vi "calibrate_handle.vi"(8 "Decimated pose (manipulator)":dbl[][][](array[numeric]) format="%#_3p", 9 "Tip offset":sgl[](array[numeric]), 11 "Light 3 pos":sgl[][](array[numeric])) -> (0 "Handle error":T1 format="%#_3g", 1 "RMS Error":dbl format="%#_3g", 3 "Handle transform":T1 format="%#_3p")   [LabVIEW 2013]
uses:
  <vilib>/Analysis/Matrix/Datatypes/RealMatrix.ctl
  <vilib>/Analysis/baseanly.llb/A x Vector.vi
  <vilib>/Analysis/baseanly.llb/Vector x A.vi
  <vilib>/Analysis/_algsub.llb/Real PseudoInverse Matrix.vi
  <vilib>/Analysis/baseanly.llb/Real A x B.vi
  <vilib>/Analysis/Matrix/Numeric/Multiply/Multiply - RM,RM.vi
  <vilib>/Analysis/NI_AALBase.lvlib
  <vilib>/Analysis/NI_AALPro.lvlib
  <vilib>/Analysis/Matrix/NI_Matrix.lvlib
panel:
  out "Calibrated central tip pos in manipulator":dbl[][](graph)
  out "L3 pos in manipulator":dbl[][](graph)
  out "Central tip pos in manipulator":dbl[][](graph)
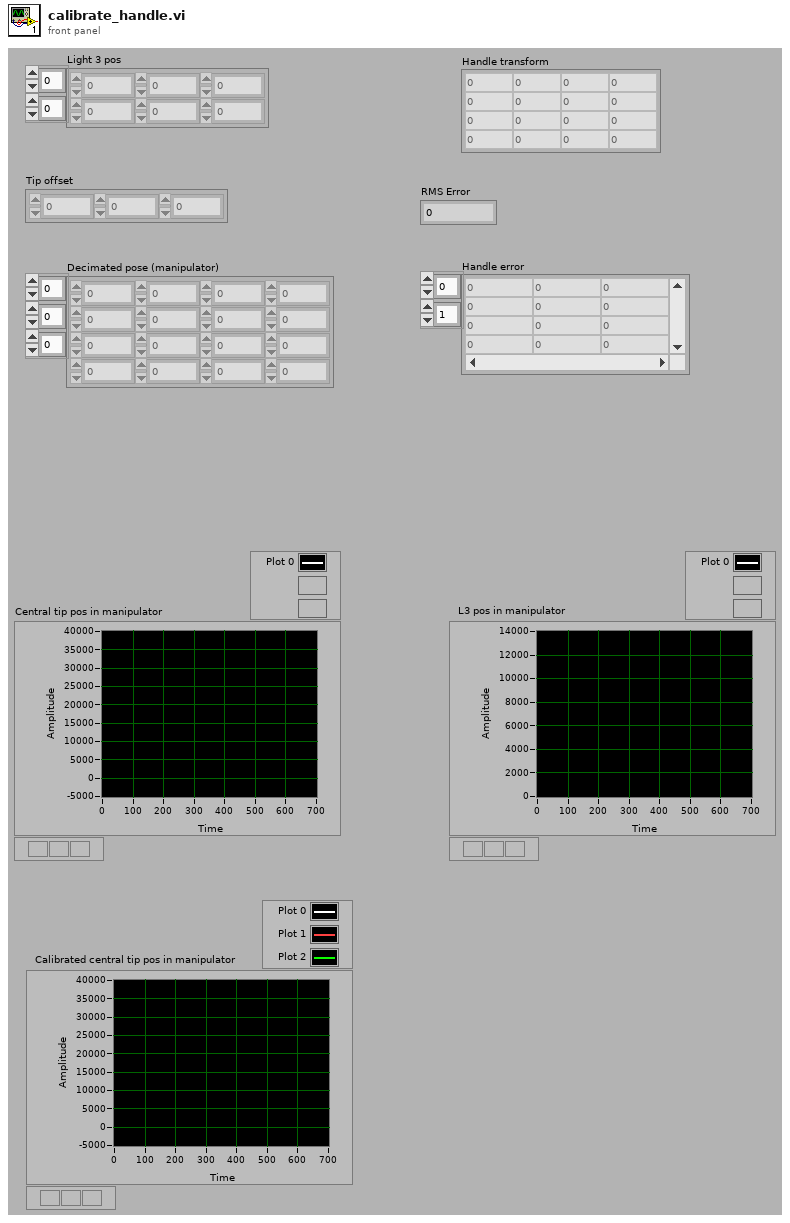
[diagram p1: front panel]
types:
  T1 = typedef "NI_Matrix.lvlib/RealMatrix.ctl" = dbl[][]
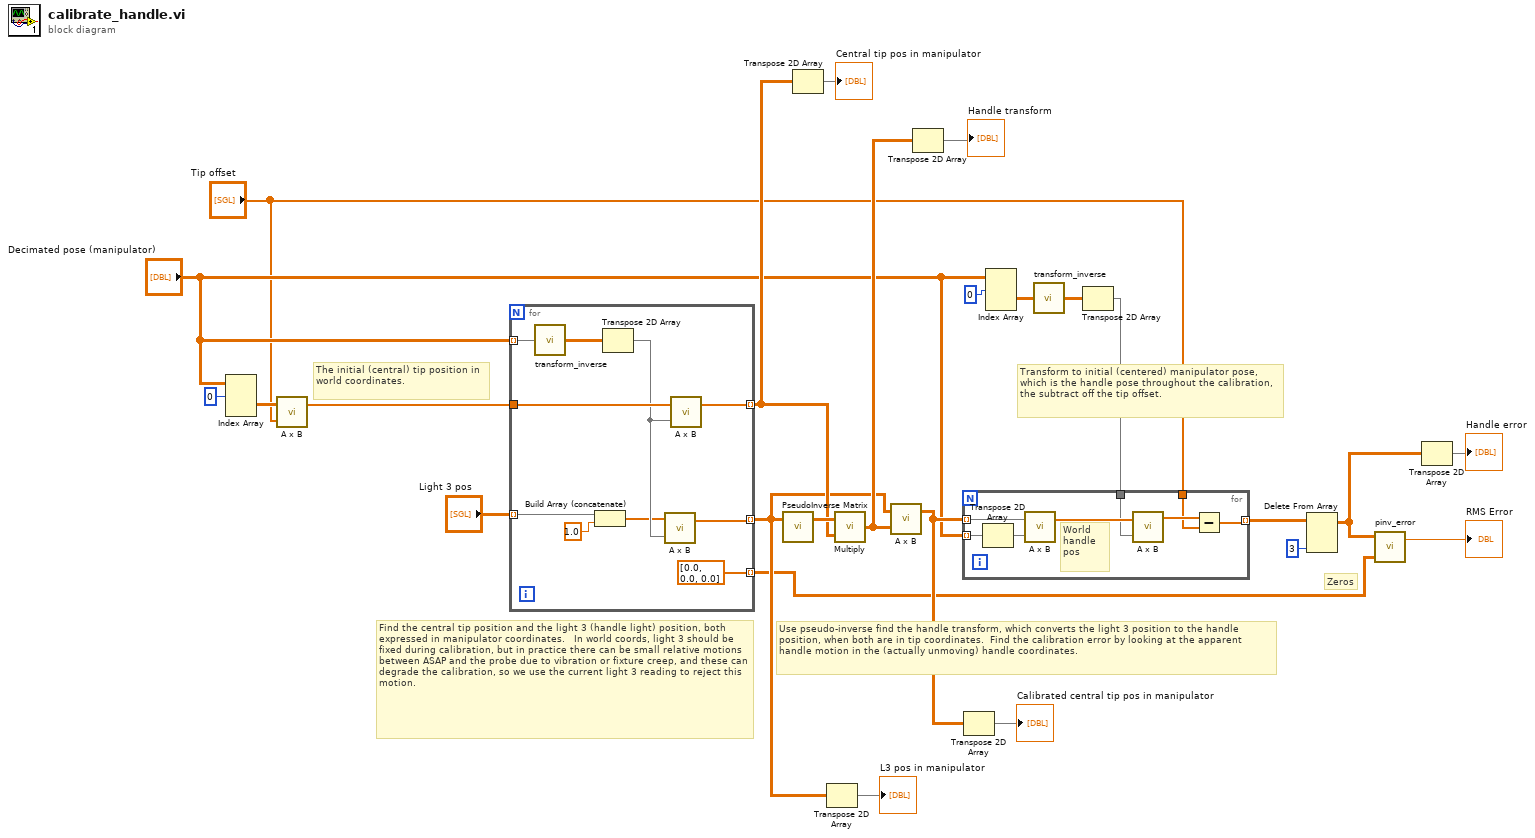
[diagram p0: block diagram]
diagram:
  # "Zeros"
  # "Use pseudo-inverse find the handle transform, which converts the light 3 position to the handle position, when both are in tip coordinates.  Find the calibration error by looking at the apparent handle motion in the (actually unmoving) handle coordinates."
  # "Transform to initial (centered) manipulator pose, which is the handle pose throughout the calibration, the subtract off the tip offset."
  # "The initial (central) tip position in world coordinates."
  # "Find the central tip position and the light 3 (handle light) position, both expressed in manipulator coordinates.   In world coords, light 3 should be fixed during calibration, but in practice there can be small relative motions between ASAP and the probe due to vibration or fixture creep, and these can degrade the calibration, so we use the current light 3 reading to reject this motion."
  n1 = Index Array(array="Decimated pose (manipulator)", index (dim 0)=0 ("index (page)")) -> (element=w5:dbl[][])  [unwired: 2 in]
  n2 = call-poly <vilib>:"A x B.vi"("Vector"="Tip offset", "A"=w5) -> ("A x Vector"=w4:dbl[])  [unwired: 1 out]
  n3 = for {
    tunnel: "Decimated pose (manipulator)" -> [w31] mode=indexing
    tunnel: [w35] -> w8 mode=indexing
    tunnel: [w34] -> w9 mode=indexing
    tunnel: w4 -> [w33]
    tunnel: [dbl[] [0.0, 0.0, 0.0] ("Tip offset")] -> w3 mode=indexing
    tunnel: "Light 3 pos" -> [w27] mode=indexing
    n4 = call "transform_inverse.vi"("Transform"=w31) -> ("Inverse transform"=w30:T1)
    n5 = Build Array (concatenate)(w27, sgl 1.0) -> (w26:sgl[])
    n6 = Transpose 2D Array(2D array=w30) -> (transposed array=w32:T1)
    n7 = call-poly <vilib>:"A x B.vi"("Matrix A"=w32, "Vector V'"=w26) -> ("V' x A"=w35:dbl[])  [unwired: 1 out]
    n8 = call-poly <vilib>:"A x B.vi"("Matrix A"=w32, "Vector V'"=w33) -> ("V' x A"=w34:dbl[])  [unwired: 1 out]
  }
  n9 = call-poly <vilib>:"PseudoInverse Matrix.vi"("Input Matrix"=w8) -> ("PseudoInverse Matrix"=w25:T1)  [unwired: 1 in, 1 out]
  n10 = Transpose 2D Array(2D array=w9) -> (transposed array=→"Central tip pos in manipulator":dbl[][])
  n11 = Transpose 2D Array(2D array=w8) -> (transposed array=→"L3 pos in manipulator":dbl[][])
  n12 = call-poly <vilib>:"Multiply.vi"("Real Matrix B"=w9, "Real Matrix A"=w25) -> ("A * B"=w21:T1)
  n13 = call-poly <vilib>:"A x B.vi"("B"=w21, "A"=w8) -> ("A x B"=w10:T1)  [unwired: 1 out]
  n14 = Transpose 2D Array(2D array=w21) -> (transposed array=→"Handle transform":T1)
  n15 = Transpose 2D Array(2D array=w10) -> (transposed array=→"Calibrated central tip pos in manipulator":T1)
  n16 = Index Array(array="Decimated pose (manipulator)", index (dim 0)=0 ("index (page)")) -> (element=w19:dbl[][])  [unwired: 2 in]
  n17 = call "transform_inverse.vi"("Transform"=w19) -> ("Inverse transform"=w18:T1)
  n18 = Transpose 2D Array(2D array=w18) -> (transposed array=w17:T1)
  n19 = for {
    tunnel: "Decimated pose (manipulator)" -> [w40] mode=indexing
    tunnel: w10 -> [w43] mode=indexing
    tunnel: [w36] -> w15 mode=indexing
    tunnel: w17 -> [w41]
    tunnel: "Tip offset" -> [w37]
    # "World handle pos"
    n20 = Transpose 2D Array(2D array=w40) -> (transposed array=w39:dbl[][])
    n21 = call-poly <vilib>:"A x B.vi"("Matrix A"=w39, "Vector V'"=w43) -> ("V' x A"=w42:dbl[])  [unwired: 1 out]
    n22 = call-poly <vilib>:"A x B.vi"("Matrix A"=w41, "Vector V'"=w42) -> ("V' x A"=w38:dbl[])  [unwired: 1 out]
    n23 = Subtract(x=w38, y=w37) -> (x-y=w36:dbl[])
  }
  n24 = Delete From Array(array=w15, index (col)=3 ("index (row)")) -> (array with subset deleted=w14:dbl[][])  [unwired: 2 in, 1 out]
  n25 = call "pinv_error.vi"("Y"=w3, "Calibrated"=w14) -> ("Error"=→"RMS Error":dbl)  [unwired: 1 in, 1 out]
  n26 = Transpose 2D Array(2D array=w14) -> (transposed array=→"Handle error":dbl[][])
